vi "test--Get Control Tags.vi"() -> ()   [LabVIEW 2021]
doc: "test vi to check the tags of the ctl files\n\n<b>Code Developed By:</b>\nTechnology Service Corporation\n1983 S Liberty Drive\nBloomington, IN 47403\nPhone: 812 558-7100\nwww.tsc.com/atcs\n\nDeveloper:\nDaniel Coons"
panel:
  out "filenames":string[](array[string])
  out "tags":string[](array[string])
  in  "Tag Name":string="button-type"
  out "error out":errorcluster
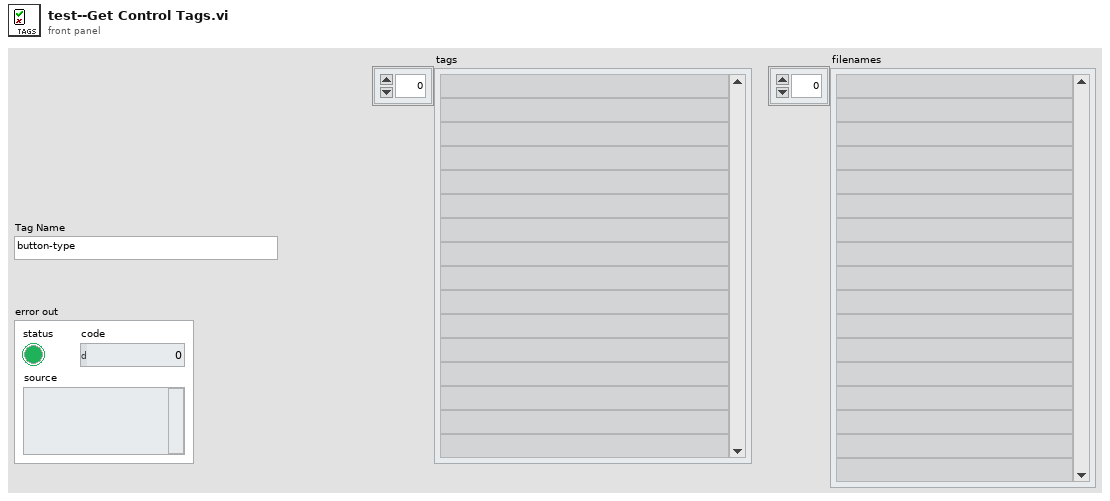
[diagram p1: front panel]
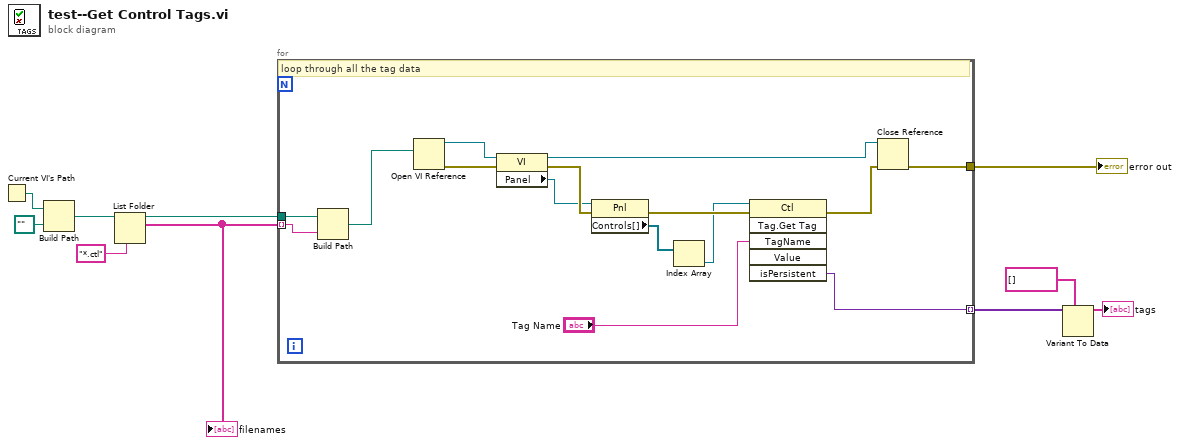
[diagram p0: block diagram]
diagram:
  n1 = Current VI's Path() -> (path=w9:path)
  n2 = Build Path(base path=w9, name or relative path=path "..") -> (appended path=w7:path)
  n3 = List Folder(path=w7, pattern="*.ctl") -> (path out=w5:path, filenames=w4:string[])  [unwired: 2 in, 2 out]
  "filenames" <- w4
  n4 = for {
    tunnel: [w19] -> w10
    tunnel: w5 -> [w15]
    tunnel: w4 -> [w14] mode=indexing
    tunnel: [w11] -> w3 mode=indexing
    # "loop through all the tag data"
    n5 = Build Path(base path=w15, name or relative path=w14) -> (appended path=w13:path)
    n6 = Open VI Reference(vi path=w13) -> (vi reference=w23:refnum<vi>, error out=w25:errorcluster)  [unwired: 5 in]
    n7 = property class="VI"(reference=w23, error in=w25) -> (reference out=w12:refnum<vi>, error out=w24:errorcluster, "Panel"=w21:refnum<vi>)
    n8 = property class="Pnl"(reference=w21, error in=w24) -> (error out=w22:errorcluster, "Controls[]"=w20:refnum<vi>[])  [unwired: 1 out]
    n9 = Index Array(array=w20) -> (element=w17:refnum<vi>)  [unwired: 1 in]
    n10 = invoke class="Ctl" method="Tag.Get Tag"(reference=w17, error in=w22, "TagName"="Tag Name") -> (error out=w18:errorcluster, "isPersistent"=w11:variant)  [unwired: 3 in, 4 out]
    n11 = Close Reference(reference=w12, error in (no error)=w18) -> (error out=w19:errorcluster)
  }
  "error out" <- w10
  n12 = Variant To Data(type=string[] [], Variant=w3) -> (data=→"tags":string[])  [unwired: 1 in, 1 out]
